vi "均匀ADC.vi"(8 "量化阶 V":dbl=0.02, 11 "输入的模拟信号取样值 V":dbl(ring)=0.075 items=["0.075"=0.075, "0.130"=0.13, "0.131"=0.131, "1.239"=1.239, "2.510"=2.51, "-2.540"=-2.54, "-2.700"=-2.7]) -> (2 "数字编码":dbl[](array[numeric]))   [LabVIEW 2020]
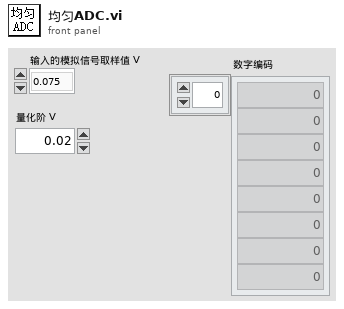
[diagram p1: front panel]
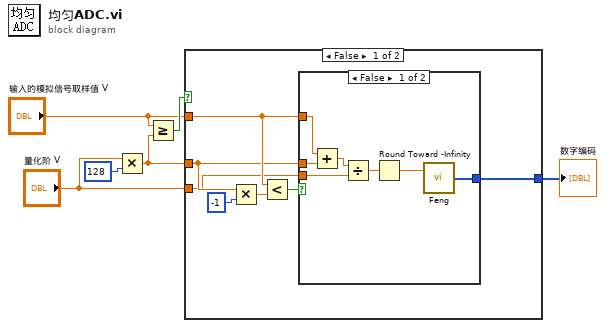
[diagram p0: block diagram]
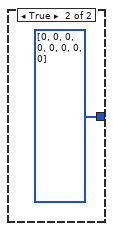
[diagram p2: hidden frame]
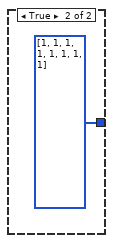
[diagram p3: hidden frame]
diagram:
  n1 = Multiply(x="量化阶 V", y=128) -> (x*y=w4:dbl)
  n2 = Greater Or Equal?(x="输入的模拟信号取样值 V", y=w4) -> (x >= y?=w5:bool)
  n3 = case shown="False" w5 {
    tunnel: [w7 i32[] [1, 1, 1, 1, 1, 1, 1, 1]] -> w2
    tunnel: w4 -> [w9 _]
    tunnel: "输入的模拟信号取样值 V" -> [w10 _]
    tunnel: "量化阶 V" -> [w8 _]
    frame False {
      n4 = Multiply(x=w9, y=-1) -> (x*y=w12:dbl)
      n5 = Less?(x=w10, y=w12) -> (x < y?=w11:bool)
      n6 = case shown="False" w11 {
        tunnel: [w14 i32[] [0, 0, 0, 0, 0, 0, 0, 0]] -> w7
        tunnel: w10 -> [w20 _]
        tunnel: w9 -> [w19 _]
        tunnel: w8 -> [w17 _]
        frame False {
          n7 = Add(x=w20, y=w19) -> (x+y=w18:dbl)
          n8 = Divide(x=w18, y=w17) -> (x/y=w16:dbl)
          n9 = Round Toward -Infinity(1:w16) -> (0:w15:dbl)
          n10 = call "Feng.vi"("decimal 2"=w15) -> ("bitstream 3"=w14:i32[])  [unwired: 1 in]
        }
        frame True {
        }
      }
    }
    frame True {
    }
  }
  "数字编码" <- w2
